vi "oa_Process Counter Data (No State).vi"(6 "state in":T1, 7 "reset":bool, 8 "error in (no error)":errorcluster, 9 "vibration signal duration [s]":dbl, 10 "tacho counts":i64[](array[numeric]), 11 "digital tach info in":T2) -> (0 "error out":errorcluster, 3 "digital tach info out":T2, 4 "state out":T1)   [LabVIEW 2017, in "SoundVib_TachProcess.lvlib"]
uses:
  <vilib>/addons/Sound and Vibration/Order Analysis/Tach Process/SoundVib_TachProcess.lvlib
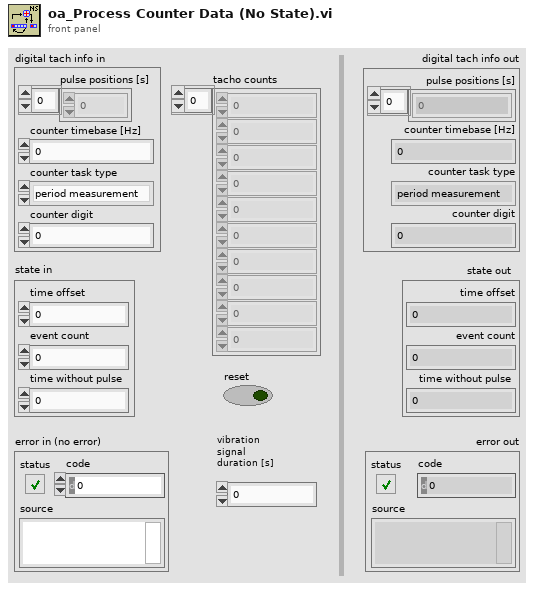
[diagram p1: front panel]
types:
  T1 = cluster{"time offset":dbl, "event count":u64, "time without pulse":ext}
  T2 = cluster{"pulse positions [s]":dbl[], "counter timebase [Hz]":dbl, "counter task type":enum16{"period measurement", "event counting"}, "counter digit":i32}
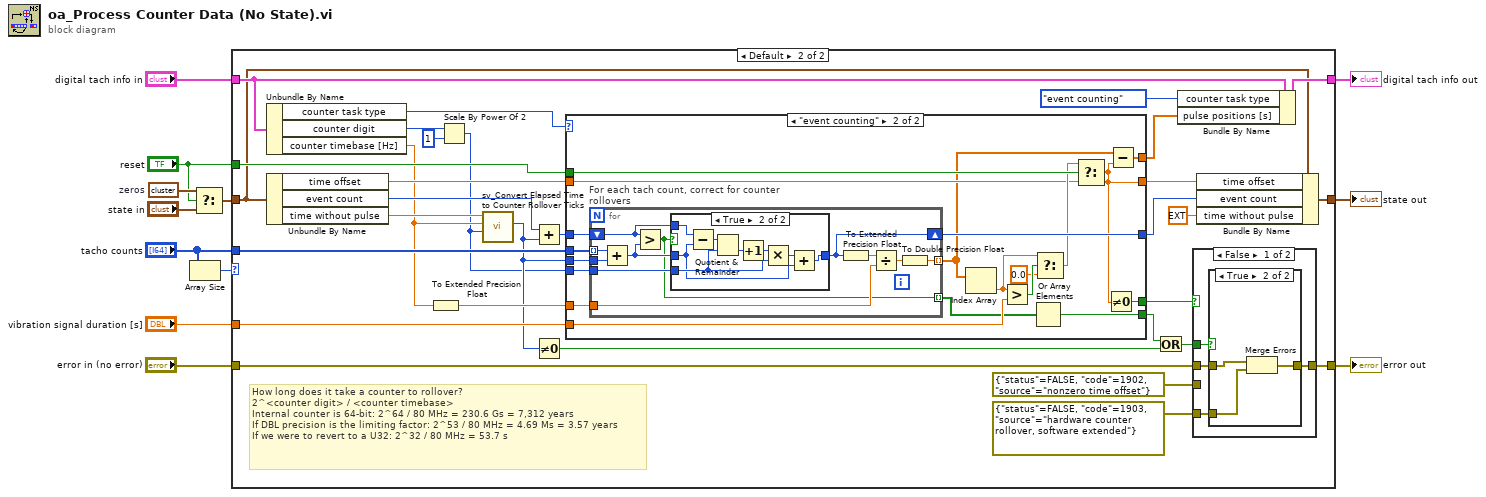
[diagram p0: block diagram]
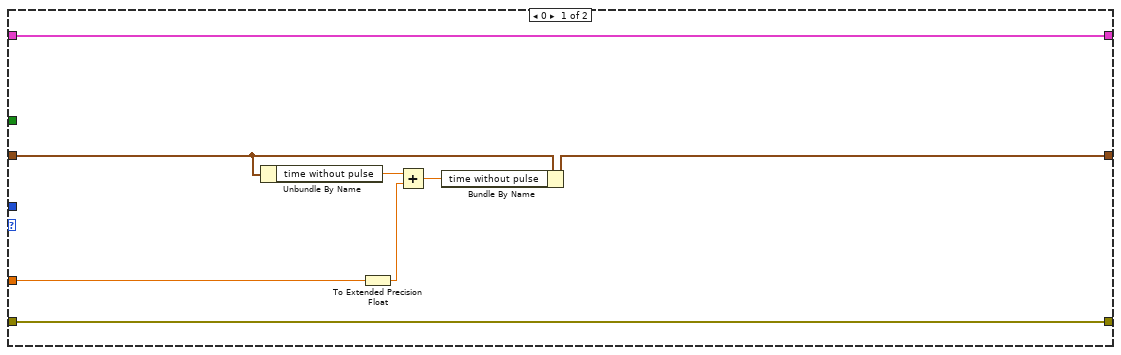
[diagram p2: hidden frame]
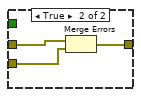
[diagram p4: hidden frame]
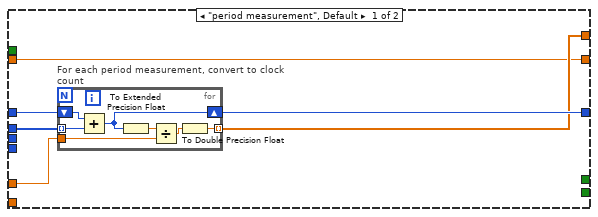
[diagram p5: hidden frame]
diagram:
  w7 = T1 {"time offset"=0.0, "event count"=0, "time without pulse"=0.0}  # zeros
  n1 = Array Size(array="tacho counts") -> (size(s)=w9:i32)
  n2 = Select(t=w7, s="reset", f="state in") -> (s? t:f=w4:T1)
  n3 = case shown="Default" w9 {
    tunnel: "digital tach info in" -> [w18 w34]
    tunnel: "vibration signal duration [s]" -> [w19 w45]
    tunnel: [w18 w47] -> w12
    tunnel: "tacho counts" -> [_ w51]
    tunnel: "reset" -> [_ w41]
    tunnel: w4 -> [w14 w33]
    tunnel: [w16 w37] -> w3
    tunnel: "error in (no error)" -> [w13 w31]
    tunnel: [w13 w30] -> w1
    frame 0 {
      n4 = Unbundle By Name(w14) -> ("time without pulse"=w17:ext)
      n5 = To Extended Precision Float(1:w19) -> (0:w20:ext)
      n6 = Add(x=w17, y=w20) -> (x+y=w15:ext)
      n7 = Bundle By Name(cluster=w14, "time without pulse"=w15) -> (w16:T1)
    }
    frame Default {
      # "How long does it take a counter to rollover?\n2^<counter digit> / <counter timebase>\nInternal counter is 64-bit: 2^64 / 80 MHz = 230.6 Gs = 7,312 years\nIf DBL precision is the limiting factor: 2^53 / 80 MHz = 4.69 Ms = 3.57 years\nIf we were to revert to a U32: 2^32 / 80 MHz = 53.7 s"
      n8 = Unbundle By Name(w34) -> ("counter task type"=w36:enum16{"period measurement", "event counting"}, "counter digit"=w35:i32, "counter timebase [Hz]"=w23:dbl)
      n9 = Unbundle By Name(w33) -> ("time offset"=w43:dbl, "event count"=w42:u64, "time without pulse"=w24:ext)
      n10 = To Extended Precision Float(1:w23) -> (0:w49:ext)
      n11 = Scale By Power Of 2(n=w35, x=u64 1) -> (x*2^n=w21:u64)
      n12 = call <vilib>:"sv_Convert Elapsed Time to Counter Rollover Ticks.vi"("counter maximum value"=w21, "counter timebase (Hz)"=w23, "elapsed time (s)"=w24) -> ("elapsed rollover ticks"=w22:u64)  [unwired: 6 in, 2 out]
      n13 = Add(x=w42, y=w22) -> (x+y=w48:u64)
      n14 = Not Equal To 0?(x=w22) -> (x != 0?=w29:bool)
      n15 = case shown="\"event counting\"" w36 {
        tunnel: [w67 w94] -> w38
        tunnel: w51 -> [w68 w90]
        tunnel: w49 -> [w66 w91]
        tunnel: w48 -> [w65 w93]
        tunnel: w22 -> [_ w89]
        tunnel: [w64 w81] -> w46
        tunnel: w21 -> [_ w92]
        tunnel: w41 -> [_ w86]
        tunnel: w45 -> [_ w88]
        tunnel: [w63 w77] -> w40
        tunnel: w43 -> [w63 w82]
        tunnel: [_ w78] -> w28
        tunnel: [_ w76] -> w32
        frame "period measurement", Default {
          n16 = for "For each period measurement, convert to clock count" {
            shift-right: [w74] -> w67
            shift-left: w65 -> [w75]
            tunnel: [w69] -> w64 mode=indexing
            tunnel: w68 -> [w73] mode=indexing
            tunnel: w66 -> [w72]
            n17 = Add(x=w75, y=w73) -> (x+y=w74:u64)
            n18 = To Extended Precision Float(1:w74) -> (0:w71:ext)
            n19 = Divide(x=w71, y=w72) -> (x/y=w70:ext)
            n20 = To Double Precision Float(number=w70) -> (double precision float=w69:dbl)
          }
        }
        frame "event counting" {
          n21 = for "For each tach count, correct for counter rollovers" {
            shift-right: [w102] -> w94
            shift-left: w93 -> [w99]
            tunnel: [w101] -> w80 mode=indexing
            tunnel: w92 -> [w100]
            tunnel: w91 -> [w103]
            tunnel: w90 -> [w98] mode=indexing
            tunnel: w89 -> [w97]
            tunnel: [w95] -> w79 mode=indexing
            n22 = Add(x=w98, y=w97) -> (x+y=w96:u64)
            n23 = Greater?(x=w99, y=w96) -> (0:w95:bool)
            n24 = case shown="True" w95 {
              tunnel: w96 -> [w106 w107]
              tunnel: [w106 w114] -> w102
              tunnel: w100 -> [_ w110]
              tunnel: w99 -> [_ w113]
              frame False {
              }
              frame True {
                n25 = Subtract(x=w113, y=w107) -> (x-y=w112:u64)
                n26 = Quotient & Remainder(x=w112, y=w110) -> (floor(x/y)=w111:u64)  [unwired: 1 out]
                n27 = Increment(x=w111) -> (x+1=w109:u64)
                n28 = Multiply(x=w109, y=w110) -> (x*y=w108:u64)
                n29 = Add(x=w108, y=w107) -> (x+y=w114:u64)
              }
            }
            n30 = To Extended Precision Float(1:w102) -> (0:w105:ext)
            n31 = Divide(x=w105, y=w103) -> (x/y=w104:ext)
            n32 = To Double Precision Float(number=w104) -> (double precision float=w101:dbl)
          }
          n33 = Index Array(array=w80) -> (element=w85:dbl)  [unwired: 1 in]
          n34 = Greater?(x=w85, y=w88) -> (0:w87:bool)
          n35 = Or Array Elements(Boolean array=w79) -> (logical OR=w78:bool)
          n36 = Select(t=w85, s=w87, f=0.0) -> (s? t:f=w83:dbl)
          n37 = Select(t=w83, s=w86, f=w82) -> (s? t:f=w77:dbl)
          n38 = Not Equal To 0?(x=w77) -> (x != 0?=w76:bool)
          n39 = Subtract(x=w80, y=w77) -> (x-y=w81:dbl[])
        }
      }
      n40 = Or(x=w28, y=w29) -> (x .or. y?=w27:bool)
      n41 = Bundle By Name(cluster=w34, "counter task type"=enum16{"period measurement", "event counting"}."event counting", "pulse positions [s]"=w46) -> (w47:T2)
      n42 = case shown="False" w32 {
        tunnel: w27 -> [w55 _]
        tunnel: [w54 w61] -> w30
        tunnel: w31 -> [w53 w62]
        tunnel: errorcluster {"status"=FALSE, "code"=1903, "source"="hardware counter rollover, software extended"} ("error in") -> [w52 _]
        tunnel: errorcluster {"status"=FALSE, "code"=1902, "source"="nonzero time offset"} ("error in") -> [_ w60]
        frame False {
          n43 = case shown="True" w55 {
            tunnel: [w56 w58] -> w54
            tunnel: w53 -> [w56 w59]
            tunnel: w52 -> [_ w57]
            frame False {
            }
            frame True {
              n44 = Merge Errors(w59, w57) -> (w58:errorcluster)
            }
          }
        }
        frame True {
          n45 = Merge Errors(w62, w60) -> (w61:errorcluster)
        }
      }
      n46 = Bundle By Name(cluster=w33, "time offset"=w40, "event count"=w38, "time without pulse"=ext 0.0 ("t")) -> (w37:T1)
    }
  }
  "digital tach info out" <- w12
  "state out" <- w3
  "error out" <- w1
